vi "LD Convert to Enum (Ch Format).vi"(10 "channel":i32=1 min=1 max=2, 11 "stringIN":string) -> (1 "index":i32, 2 "ch2form":T1(ring), 3 "ch1form":enum16{"X", "R", "X Noise", "Aux 1", "Aux 2"}(ring))   [LabVIEW 2017, in "SR830.lvlib"]
uses:
  SR830.lvlib
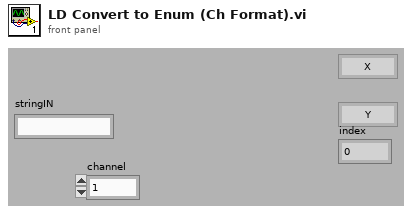
[diagram p1: front panel]
types:
  T1 = enum16{"Y", "Theta", "Y Noise", "Aux 3", "Aux 4"}
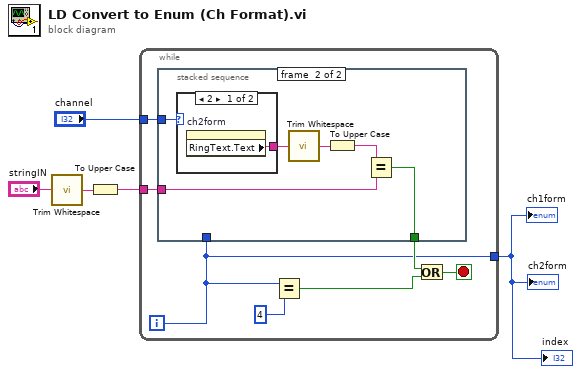
[diagram p0: block diagram]
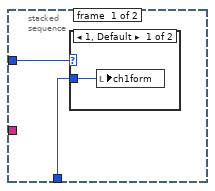
[diagram p2: hidden frame]
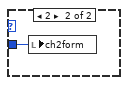
[diagram p3: hidden frame]
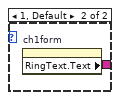
[diagram p4: hidden frame]
diagram:
  n1 = call <vilib>:"Trim Whitespace.vi"("string"="stringIN") -> ("trimmed string"=w3:string)  [unwired: 1 in]
  n2 = To Upper Case(1:w3) -> (0:w2:string)
  n3 = while {
    tunnel: "channel" -> [w12]
    tunnel: w2 -> [w11]
    tunnel: [w6] -> w1
    i -> [w6]
    stop <- w9 stop-if-true
    n4 = stacked-sequence {
      tunnel: w6 -> [w14 _]
      tunnel: w12 -> [w13 w17]
      tunnel: w11 -> [_ w19]
      tunnel: [_ w18] -> w10
      frame #0 {
        n5 = case shown="1, Default" w13 {
          tunnel: w14 -> [w15 w16]
          frame 1, Default {
            n6 = local write "ch1form"(w15) -> ()
          }
          frame 2 {
            n7 = local write "ch2form"(w16) -> ()
          }
        }
      }
      frame #1 {
        n8 = case shown="2" w17 {
          tunnel: [w23 w24] -> w21
          frame 2 {
            n9 = property on="ch2form" class="Enum (strict)"() -> ("RingText.Text"=w23:string)  [unwired: 2 in, 2 out]
          }
          frame 1, Default {
            n10 = property on="ch1form" class="Enum (strict)"() -> ("RingText.Text"=w24:string)  [unwired: 2 in, 2 out]
          }
        }
        n11 = call <vilib>:"Trim Whitespace.vi"("string"=w21) -> ("trimmed string"=w22:string)  [unwired: 1 in]
        n12 = To Upper Case(1:w22) -> (0:w20:string)
        n13 = Equal?(x=w20, y=w19) -> (x = y?=w18:bool)
      }
    }
    n14 = Equal?(x=w6, y=4) -> (x = y?=w7:bool)
    n15 = Or(x=w10, y=w7) -> (x .or. y?=w9:bool)
  }
  "ch1form" <- w1
  "ch2form" <- w1
  "index" <- w1
